vi "Receive Menu Selection Event.vi"(8 "error in (no error)":errorcluster, 10 "MenuSelectionMsg":refnum<class "MenuSelectionMsg.lvclass">, 11 "ConcreteViewModel in":refnum<class "ConcreteViewModel.lvclass">) -> (0 "error out":errorcluster, 3 "ConcreteViewModel out":refnum<class "ConcreteViewModel.lvclass">)   [LabVIEW 2018, in "TopLevelApplication.lvlib" / "ConcreteViewModel.lvclass"]
doc: "<License>\nCopyright © 2017 Composed Systems, LLC | All rights reserved\nwww.composed.io\n\nAuthor: Ethan Stern <ethan.stern@composed.io>\n\nThis software is provided \"AS IS\" WITHOUT WARRANTIES, either express or implied, AND IS FOR EDUCATIONAL PURPOSES ONLY.\n</License>"
uses:
  ConcreteViewModel.lvclass
  Source/DialogBox/OneButtonDialogBox/OneButtonDialogBox.lvclass
  modules/mva-viewable/Source/ActorEvents/IEventAggregator Messages/MenuSelectionMsg/MenuSelectionMsg.lvclass
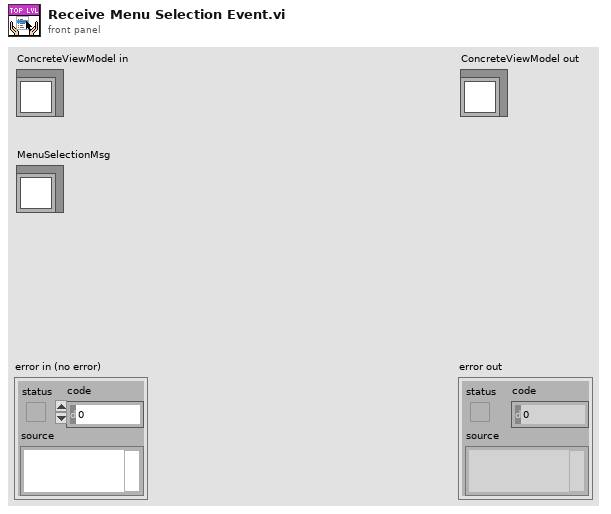
[diagram p1: front panel]
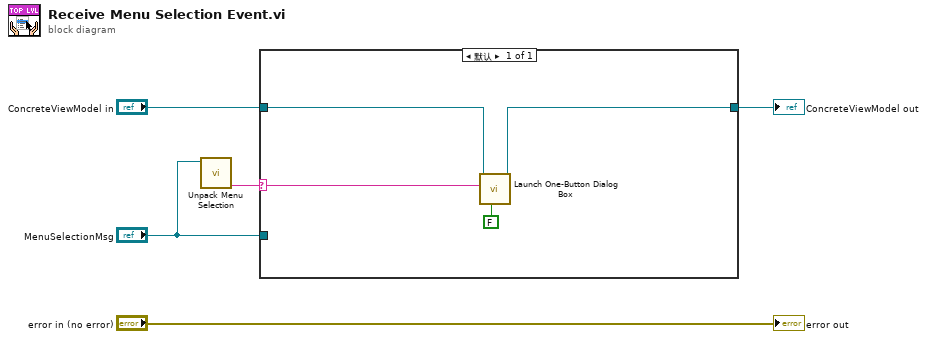
[diagram p0: block diagram]
diagram:
  n1 = call "Unpack Menu Selection.vi"("MenuSelectionMsg"="MenuSelectionMsg") -> ("Item Tag"=w1:string)  [unwired: 5 in, 5 out]
  n2 = case shown="默认" w1 {
    selector: w1 -> [w8]
    tunnel: "MenuSelectionMsg" -> [_]
    tunnel: "ConcreteViewModel in" -> [w7]
    tunnel: [w6] -> w3
    frame 默认 {
      n3 = call "Launch One-Button Dialog Box.vi"("Modal? (T)"=FALSE, "Message Text"=w8, "Dialog Launcher"=w7) -> ("Dialog Launcher Out"=w6:refnum<class "ConcreteViewModel.lvclass">)  [unwired: 7 in, 1 out]
    }
  }
  "ConcreteViewModel out" <- w3
  "error out" <- "error in (no error)"
